vi "Scripting_UpdateProtectedClassData.vi"(7 "AppRef":refnum<vi>, 8 "error in (no error)":errorcluster, 10 "NewBaseAttribute":path, 11 "BaseAttribute":path) -> (0 "error out":errorcluster, 3 "BaseAttributeReference":refnum<vi>)   [LabVIEW 2012]
uses:
  <vilib>/Utility/miscctls.llb/LVPointTypeDef.ctl
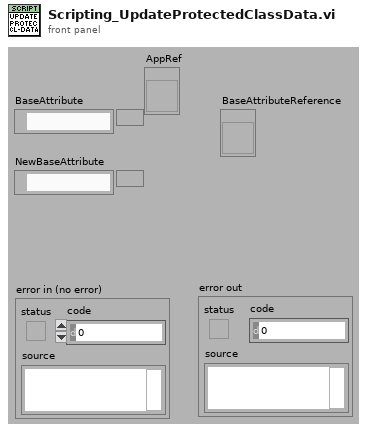
[diagram p1: front panel]
types:
  T1 = typedef "LVPointTypeDef.ctl" = cluster{"Horizontal":i16, "Vertical":i16}
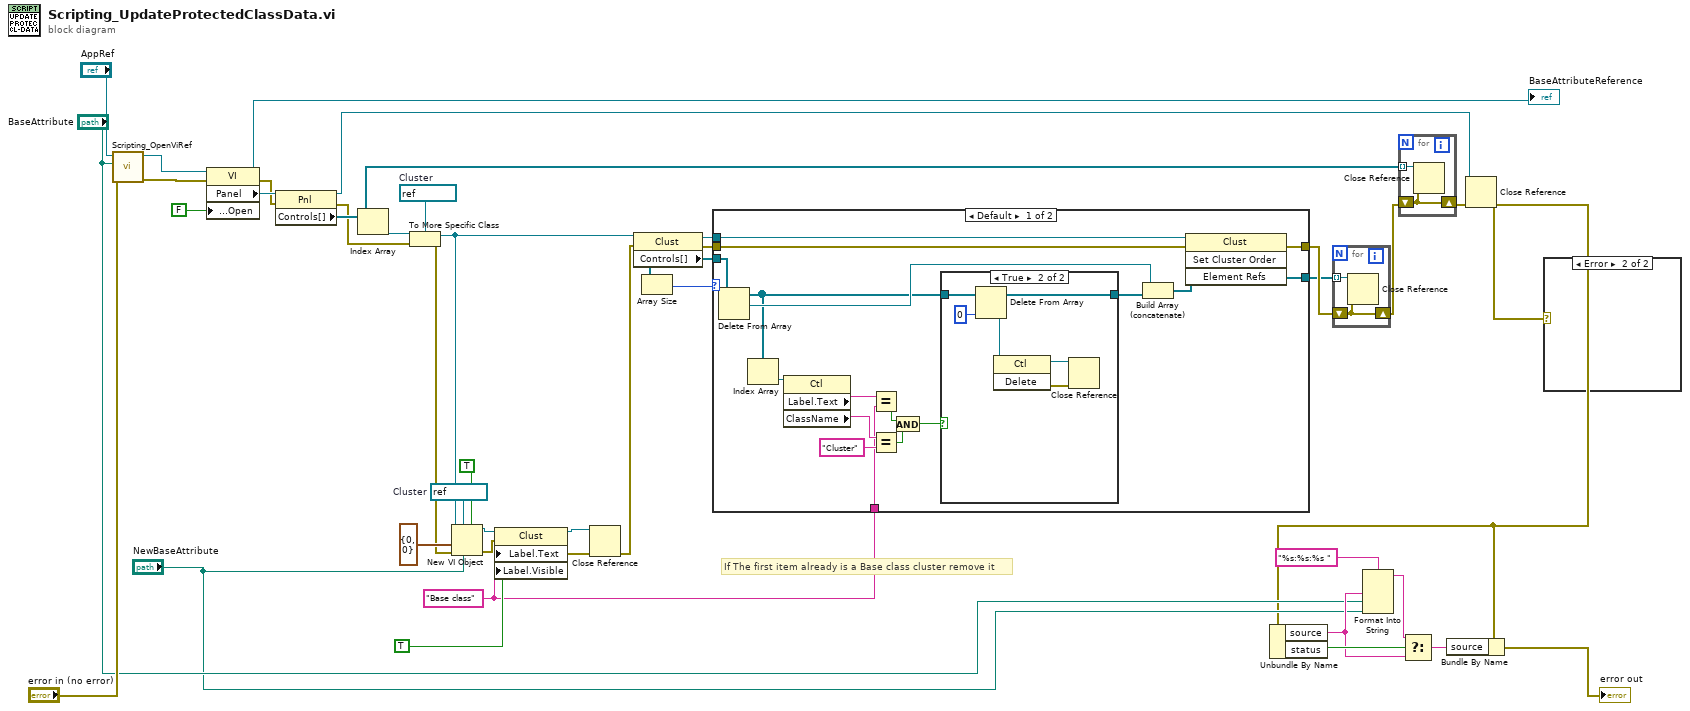
[diagram p0: block diagram]
diagram:
  w13 = "Base class" ("Label.Text")
  w23 = refnum<vi> refnum  # Cluster
  w17 = refnum<vi> refnum  # Cluster
  # "If The first item already is a Base class cluster remove it"
  n1 = call <resource>:"Scripting_OpenViRef.vi"("error in"="error in (no error)", "ViPath/ViName/Viref"="BaseAttribute", "AppRef"="AppRef") -> ("error out"=w21:errorcluster, "vi reference"=w20:refnum<vi>)  [unwired: 6 in, 1 out]
  n2 = property class="VI"(reference=w20, error in=w21, "Front Panel.Open"=FALSE ("Front Panel Window:Open")) -> (reference out=→"BaseAttributeReference":refnum<vi>, error out=w14:errorcluster, "Panel"=w15:refnum<vi>)
  n3 = property class="Pnl"(reference=w15, error in=w14) -> (reference out=w19:refnum<vi>, error out=w18:errorcluster, "Controls[]"=w38:refnum<vi>[])
  n4 = Index Array(array=w38) -> (element=w16:refnum<vi>)  [unwired: 1 in]
  n5 = To More Specific Class(target class=w17, reference=w16, error in=w18) -> (specific class reference=w31:refnum<vi>, error out=w25:errorcluster)
  n6 = New VI Object(vi object class=w23, auto wire? (F)=TRUE, owner refnum=w31, position/next to=T1 {"Horizontal"=0, "Vertical"=0} ("relative position/next to refnum"), 6:"NewBaseAttribute", 8:w25) -> (object refnum=w28:refnum<vi>, 0:w27:errorcluster)  [unwired: 2 in]
  n7 = property class="Clust"(reference=w28, error in=w27, "Label.Text"=w13, "Label.Visible"=TRUE ("Label.Visible(True)")) -> (reference out=w30:refnum<vi>, error out=w26:errorcluster)
  n8 = Close Reference(reference=w30, error in (no error)=w26) -> (error out=w32:errorcluster)
  n9 = property class="Clust"(reference=w31, error in=w32) -> (reference out=w34:refnum<vi>, error out=w33:errorcluster, "Controls[]"=w4:refnum<vi>[])
  n10 = Array Size(array=w4) -> (size(s)=w3:i32)
  n11 = case shown="Default" w3 {
    tunnel: [w58 w67] -> w36
    tunnel: [w57 w66] -> w35
    tunnel: w34 -> [w56 _]
    tunnel: w33 -> [w55 w67]
    tunnel: w13 -> [w49 _]
    tunnel: w4 -> [w43 w66]
    frame Default {
      n12 = Delete From Array(array=w43) -> (deleted portion=w54:refnum<vi>, array with subset deleted=w45:refnum<vi>[])  [unwired: 2 in]
      n13 = Index Array(array=w45) -> (element=w53:refnum<vi>)  [unwired: 1 in]
      n14 = property class="Ctl"(reference=w53) -> ("Label.Text"=w50:string, "ClassName"=w52:string)  [unwired: 1 in, 2 out]
      n15 = Equal?(x=w50, y=w49) -> (x = y?=w48:bool)
      n16 = Equal?(x=w52, y="Cluster") -> (x = y?=w47:bool)
      n17 = And(x=w48, y=w47) -> (x .and. y?=w46:bool)
      n18 = case shown="True" w46 {
        tunnel: w45 -> [w59 w65]
        tunnel: [w59 w63] -> w44
        frame False {
        }
        frame True {
          n19 = Delete From Array(array=w65, index=0) -> (deleted portion=w62:refnum<vi>, array with subset deleted=w63:refnum<vi>[])  [unwired: 1 in]
          n20 = invoke class="Ctl" method="Delete"(reference=w62) -> (reference out=w60:refnum<vi>, error out=w61:errorcluster)  [unwired: 2 in, 1 out]
          n21 = Close Reference(reference=w60, error in (no error)=w61) -> ()  [unwired: 1 out]
        }
      }
      n22 = Build Array (concatenate)(w54, w44) -> (w57:refnum<vi>[])
      n23 = invoke class="Clust" method="Set Cluster Order"(reference=w56, error in=w55, "Element Refs"=w57) -> (error out=w58:errorcluster)  [unwired: 1 in, 3 out]
    }
    frame ..1 {
    }
  }
  n24 = for {
    tunnel: w35 -> [w69] mode=indexing
    shift-right: [w68] -> w37
    shift-left: w36 -> [w68]
    n25 = Close Reference(reference=w69, error in (no error)=w68) -> ()  [unwired: 1 out]
  }
  n26 = for {
    tunnel: w38 -> [w71] mode=indexing
    shift-right: [w70] -> w40
    shift-left: w37 -> [w70]
    n27 = Close Reference(reference=w71, error in (no error)=w70) -> ()  [unwired: 1 out]
  }
  n28 = Close Reference(reference=w19, error in (no error)=w40) -> (error out=w2:errorcluster)
  n29 = Unbundle By Name(w2) -> ("source"=w8:string, "status"=w12:bool)
  n30 = Format Into String(format string="%s:%s:%s ", w8, "BaseAttribute", "NewBaseAttribute") -> (resulting string=w10:string)  [unwired: 2 in, 1 out]
  n31 = Select(t=w10, s=w12, f=w8) -> (s? t:f=w9:string)
  n32 = Bundle By Name(cluster=w2, "source"=w9) -> (→"error out":errorcluster)
  n33 = case shown="Error" w2 {
    frame No Error {
    }
    frame Error {
    }
  }
